vi "Main.vi"() -> ()   [LabVIEW 2022 SP3, in "Application.lvlib"]
doc: "This VI is the main application VI in the DQMH project template. This application VI is implemented as a simple state machine, which communicates with two different DQMH modules.\n_____\nBased on DQMH Project Template 7.0.1.1316."
uses:
  Application.lvlib
  Application Data--cluster.ctl
  State--enum.ctl
  <vilib>/Utility/error.llb/DialogType.ctl
  <vilib>/MakerHub/LINX/Public/Utilities/Open Local.vi
  HW-210/HW-210_dqmh.lvlib
  BME680/BME680_dqmh.lvlib
  Motor/Motor.lvlib
  <vilib>/MakerHub/LINX/LMH-LINX.lvlib
panel:
  in  "Boolean":bool
  in  "About DQMH":bool
  out "version":string
  in  "Hide BME680 Module":bool
  in  "Show BME680 Module":bool
  in  "Hide HW-210 Module":bool
  in  "Show HW-210 Module":bool
  in  "Stop HW-210 Module":bool
  in  "Stop BME680 Module":bool
  in  "Start BME680 Module":bool
  out "Active HW-210 Modules":string[](array[string])
  in  "Select HW-210 Module Instance":i32(ring)=-1 items=["All"=-1, "1"=1]
  out "BME680 Running?":bool
  out "Status":string
  # "This top-level application allows you to launch and control a singleton module, and multiple instances of a cloneable module."
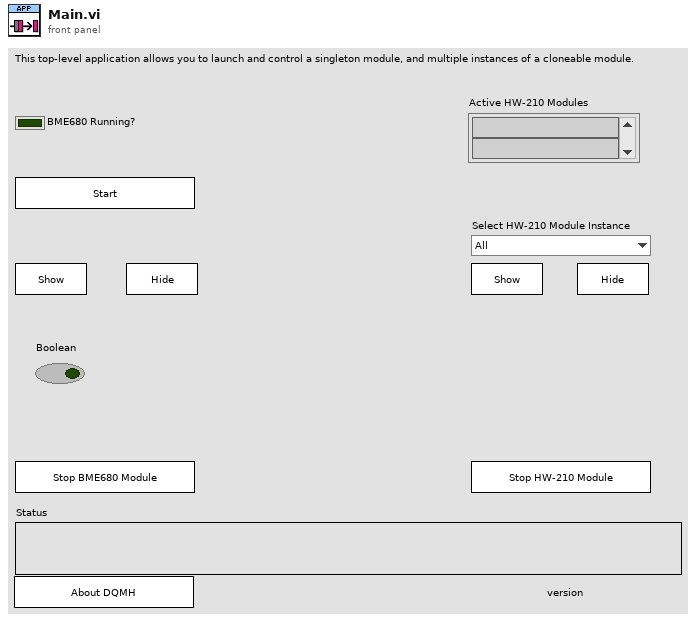
[diagram p1: front panel]
types:
  T1 = typedef "Application.lvlib/State--enum.ctl" = enum16{"Initialize", "Initialize Panel", "UI Interlocks", "Update Status", "Wait for Event", "Exit"}
  T2 = typedef "Application.lvlib/Application Data--cluster.ctl" = cluster{"Status":string, "Singleton Controls":refnum<vi>[], "Cloneable Controls":refnum<vi>[], "Module Ring Value":i32}
  T3 = typedef "Motor.lvlib/Broadcast Events--cluster.ctl" = cluster{"Module Did Init":refnum<user-event>, "Status Updated":refnum<user-event>, "Error Reported":refnum<user-event>, "Module Did Stop":refnum<user-event>, "Update Module Execution Status":refnum<user-event>, "Linx":refnum<user-event>}
  T4 = typedef "HW-210_dqmh.lvlib/Broadcast Events--cluster.ctl" = cluster{"Module Did Init":refnum<user-event>, "Status Updated":refnum<user-event>, "Error Reported":refnum<user-event>, "Module Did Stop":refnum<user-event>, "Update Module Execution Status":refnum<user-event>, "Linx":refnum<user-event>}
  T5 = typedef "BME680_dqmh.lvlib/Broadcast Events--cluster.ctl" = cluster{"Module Did Init":refnum<user-event>, "Status Updated":refnum<user-event>, "Error Reported":refnum<user-event>, "Module Did Stop":refnum<user-event>, "Update Module Execution Status":refnum<user-event>, "Linx":refnum<user-event>}
  T6 = enum8{"Enabled", "Disabled", "Disabled and Grayed Out"}
  T7 = typedef "LMH-LINX.lvlib/LINX Ref.ctl" = cluster{"IO":T8, "Interface":T9, "LINX Device Config":T10}
  T8 = typedef "LMH-LINX.lvlib/Platform.ctl" = enum16{"Remote", "Local"}
  T9 = typedef "LMH-LINX.lvlib/Interface.ctl" = enum16{"Serial", "TCP"}
  T10 = typedef "LMH-LINX.lvlib/Device.lvlib/LINX Device Config.ctl" = cluster{"Interface":T9, "COM Port":refnum<visa-resource-name>, "TCP Configuration":T11, "Device Family":u8, "Device ID":u8, "Device Name":string, "TCP Ref":refnum<k5>, "Channels":T12}
  T11 = typedef "LMH-LINX.lvlib/Device.lvlib/TCP Config.ctl" = cluster{"IP Address":string, "Port":u16}
  T12 = typedef "LMH-LINX.lvlib/Channels.ctl" = cluster{"DI":u8[], "DO":u8[], "AI":u8[], "AO":u8[], "PWM":u8[], "QE":u8[], "UART":u8[], "I2C 2":u8[], "SPI":u8[], "CAN":u8[], "Servo":u8[], "AI Ref (V)":dbl, "AI Resolution (Bits)":u8, "AO Ref (V)":dbl, "AO Resolution (Bits)":u8}
  T13 = typedef "DialogType.ctl" = u16
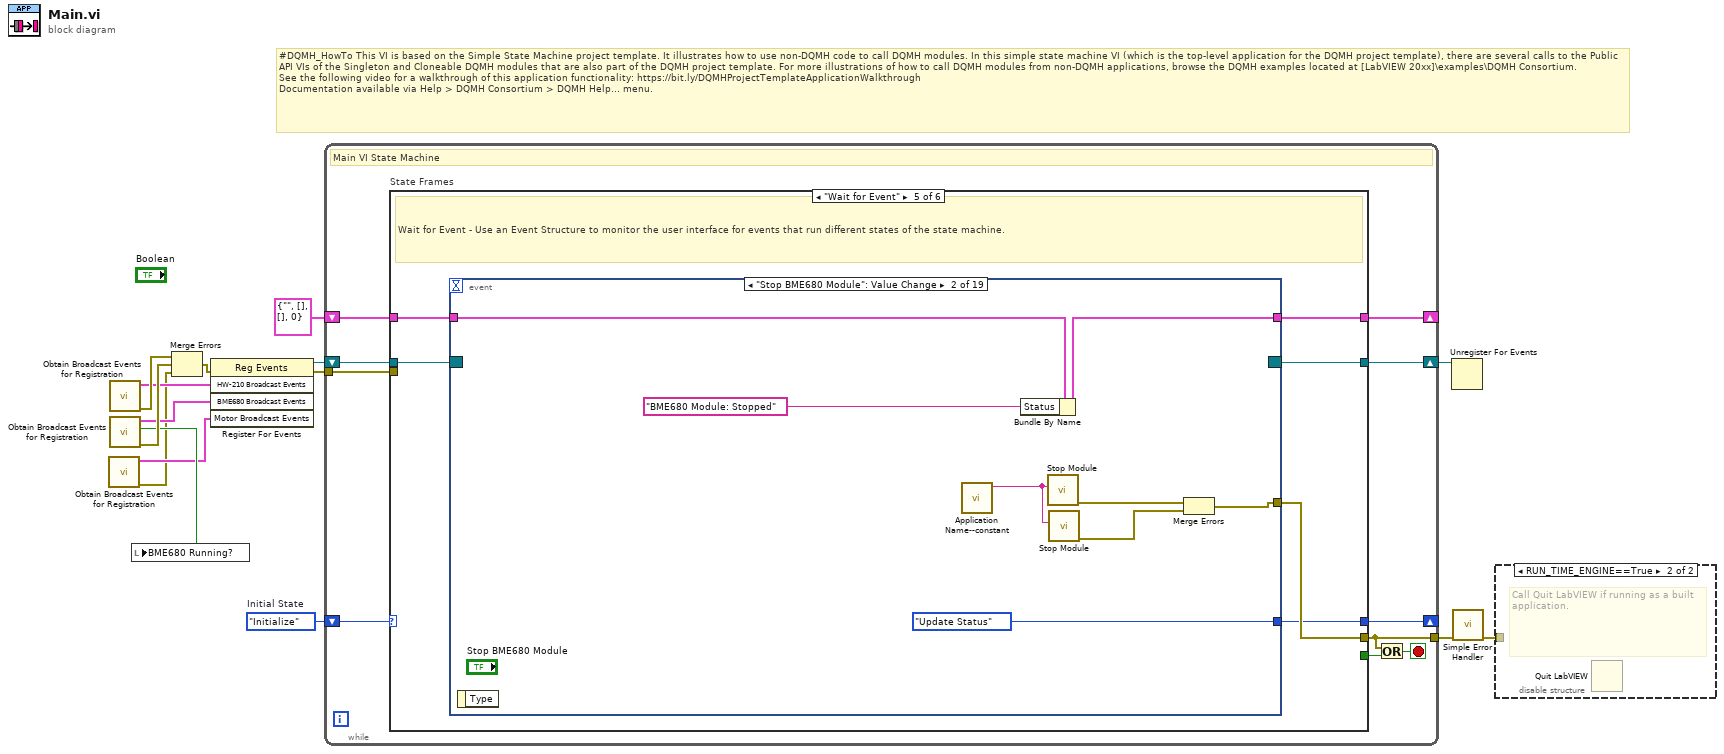
[diagram p0: block diagram]
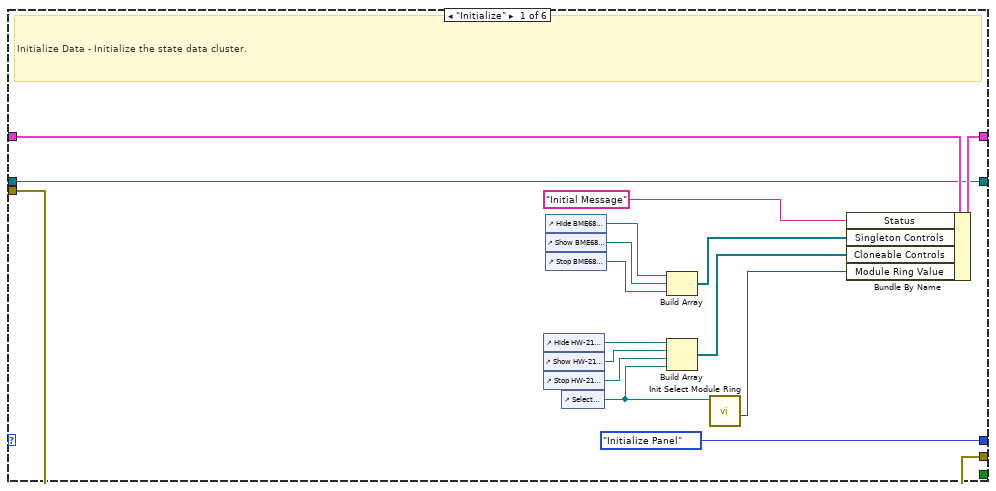
[diagram p2: hidden frame]
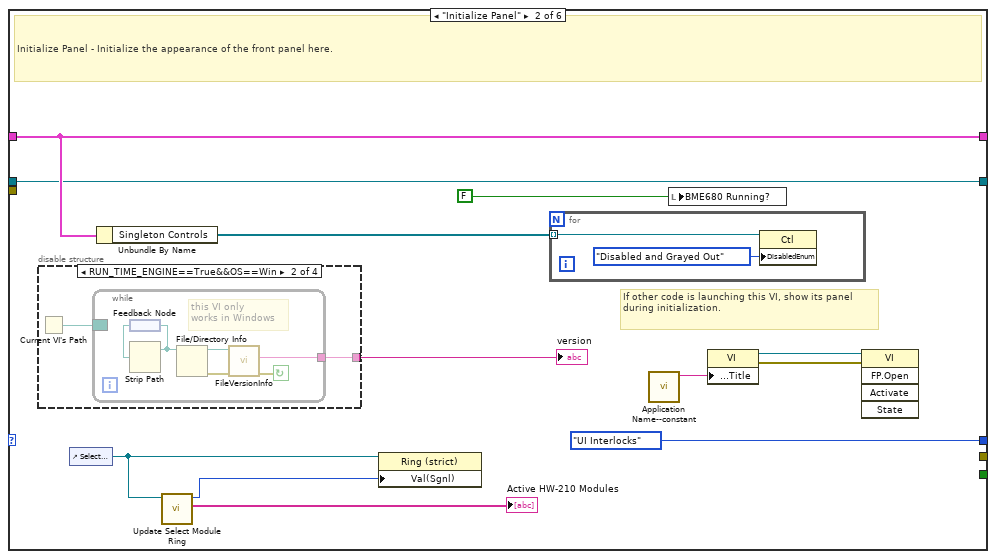
[diagram p3: hidden frame]
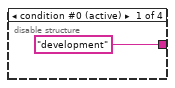
[diagram p4: hidden frame]
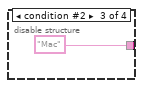
[diagram p5: hidden frame]
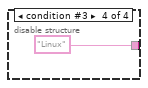
[diagram p6: hidden frame]
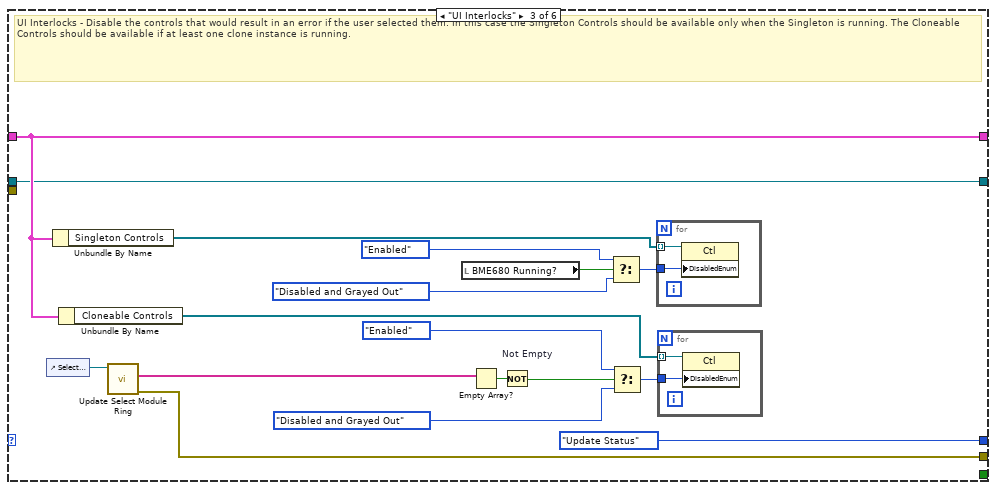
[diagram p7: hidden frame]
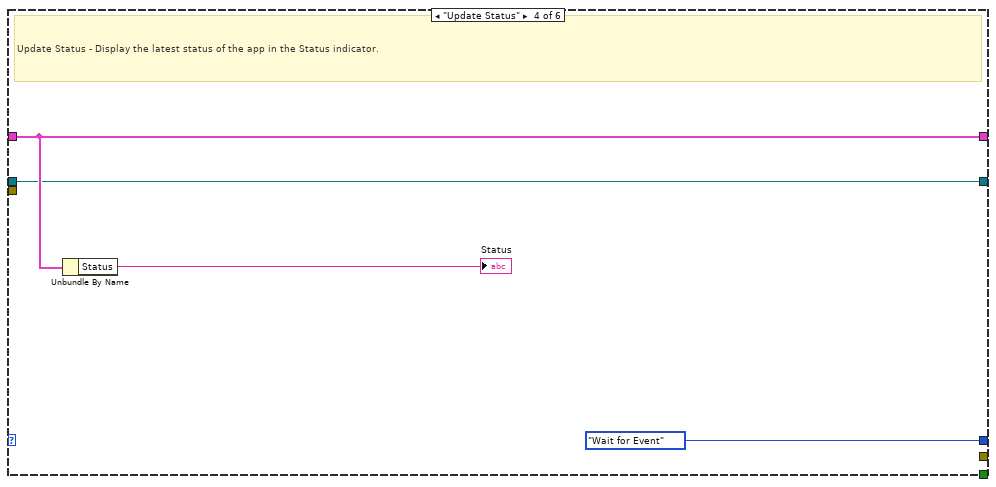
[diagram p8: hidden frame]
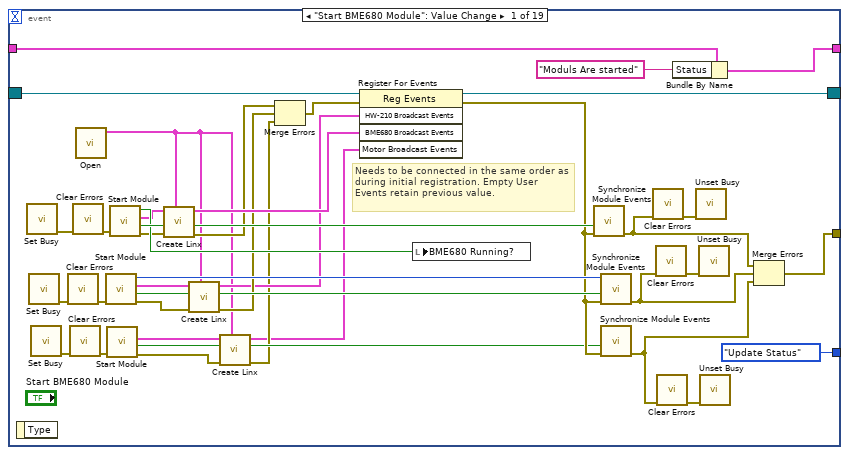
[diagram p9: hidden frame]
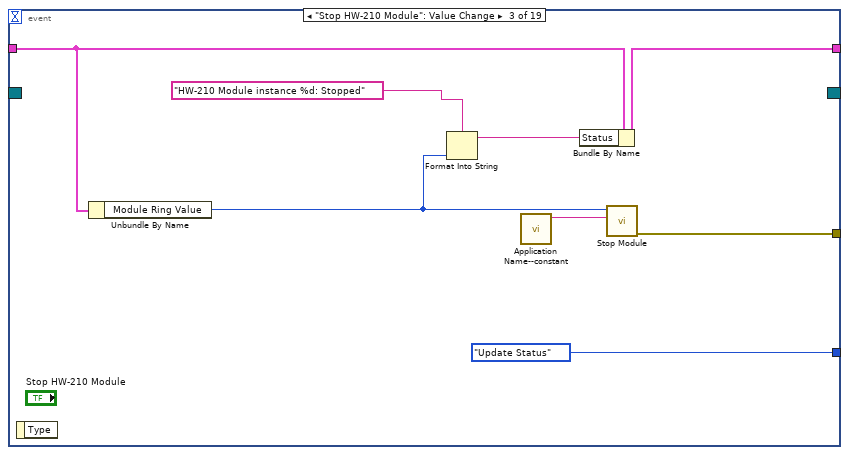
[diagram p10: hidden frame]
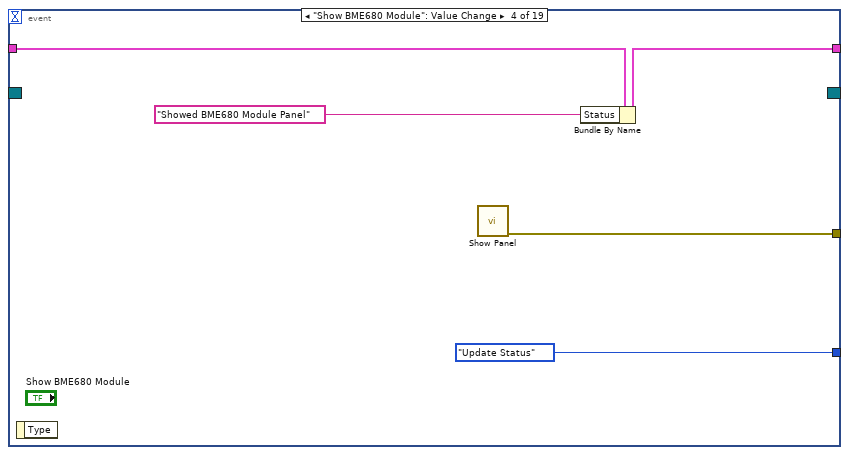
[diagram p11: hidden frame]
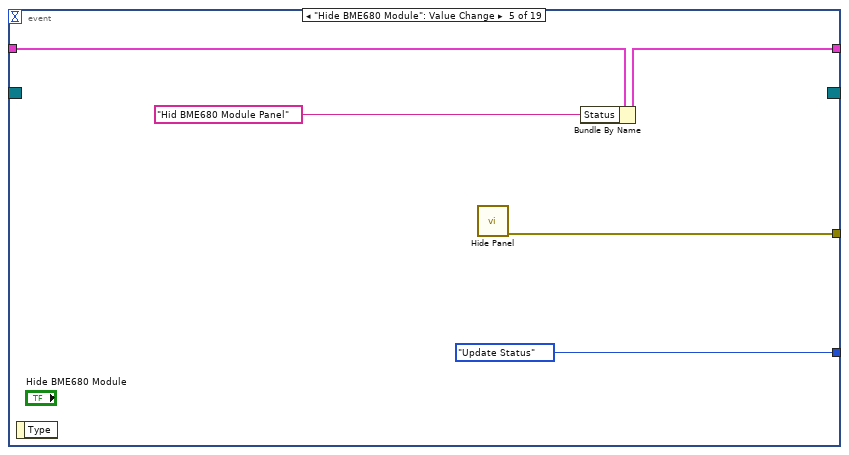
[diagram p12: hidden frame]
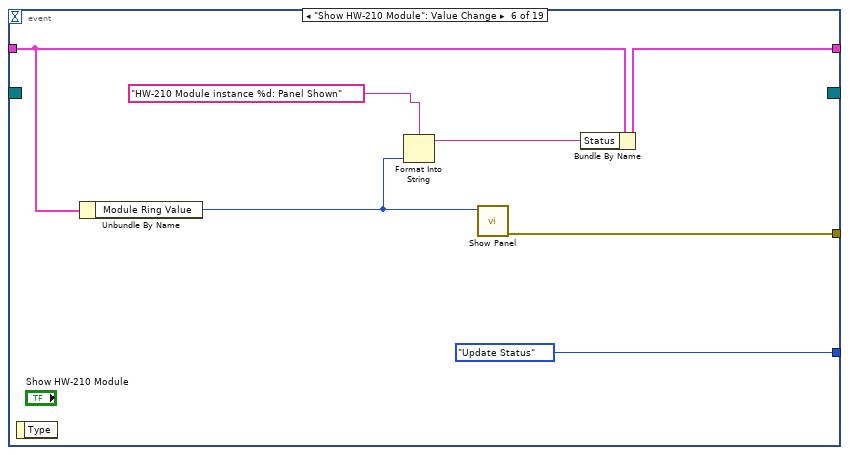
[diagram p13: hidden frame]
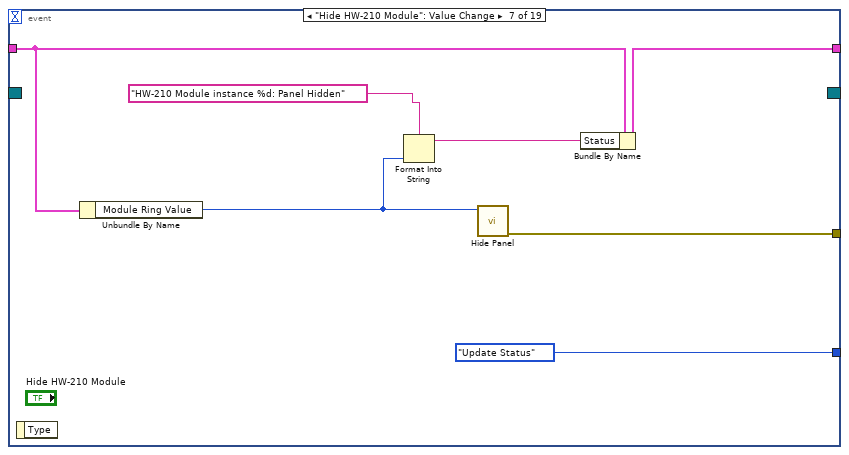
[diagram p14: hidden frame]
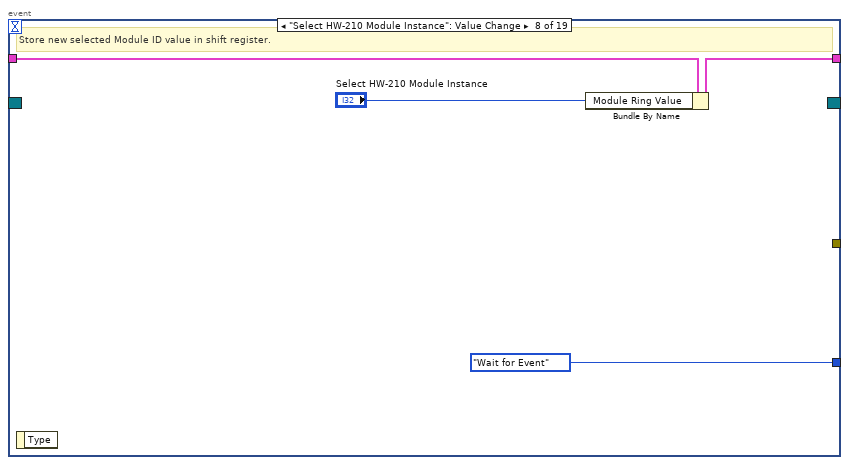
[diagram p15: hidden frame]
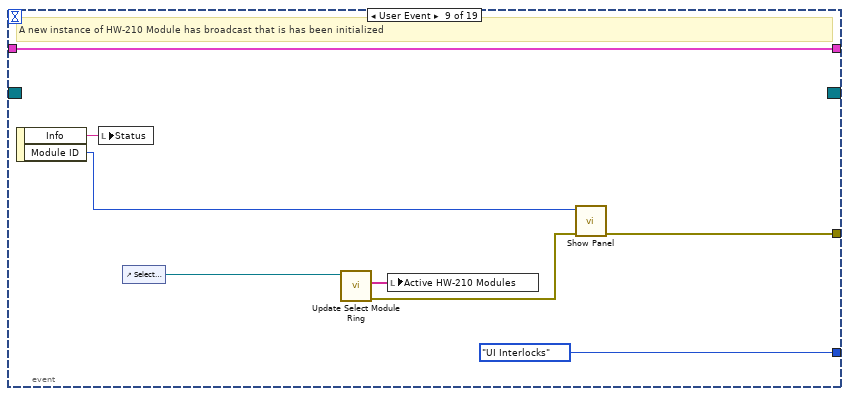
[diagram p16: hidden frame]
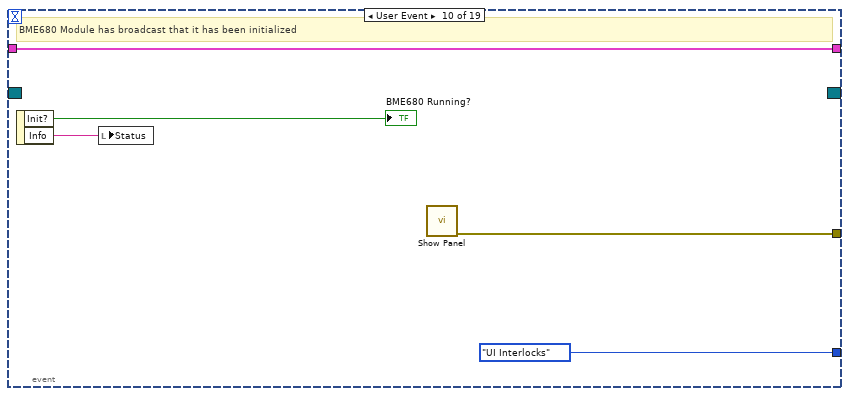
[diagram p17: hidden frame]
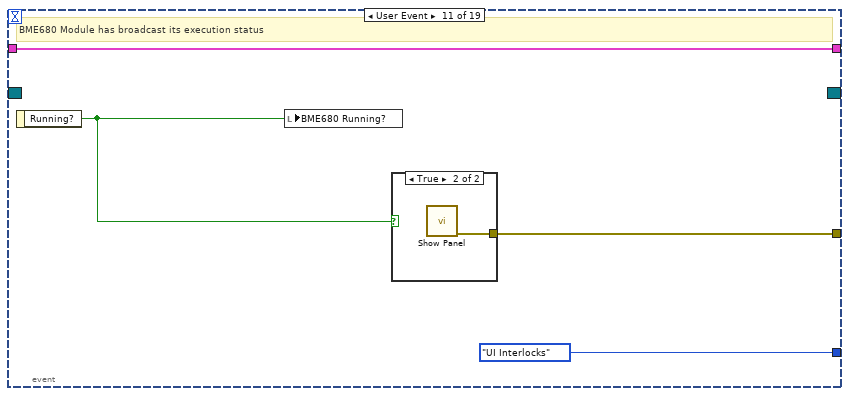
[diagram p18: hidden frame]
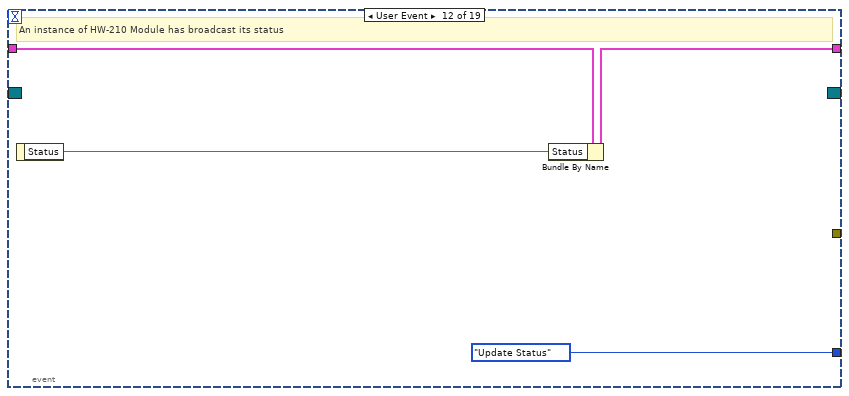
[diagram p20: hidden frame]
diagram:
  w6 = State--enum."Initialize"  # Initial State
  # "#DQMH_HowTo This VI is based on the Simple State Machine project template. It illustrates how to use non-DQMH code to call DQMH modules. In this simple state machine VI (which is the top-level application for the DQMH project template), there are several calls to the Public API VIs of the Singleton and Cloneable DQMH modules that are also part of the DQMH project template. For more illustrations of how to call DQMH modules from non-DQMH applications, browse the DQMH examples located at [LabVIEW 20xx]\\examples\\DQMH Consortium.\nSee the following video for a walkthrough of this application functionality: https://bit.ly/DQMHProjectTemplateApplicationWalkthrough\nDocumentation available via Help > DQMH Consortium > DQMH Help... menu."
  n1 = call "Obtain Broadcast Events for Registration.vi"() -> ("error out"=w1:errorcluster, "Motor Broadcast Events"=w2:T3)  [unwired: 9 in, 1 out]
  n2 = call "Obtain Broadcast Events for Registration.vi"() -> ("error out"=w11:errorcluster, "HW-210 Broadcast Events"=w8:T4)  [unwired: 9 in, 1 out]
  n3 = call "Obtain Broadcast Events for Registration.vi"() -> ("error out"=w10:errorcluster, "Already running?"=w3:bool, "BME680 Broadcast Events"=w7:T5)  [unwired: 9 in]
  n4 = local write "BME680 Running?"(w3) -> ()
  n5 = Merge Errors(w11, w10, w1) -> (w12:errorcluster)
  n6 = register-events(error in=w12, w8, w7, w2) -> (reference out=w5:refnum<event-registration>, error out=w13:errorcluster)  [unwired: 1 in]
  n7 = while {
    shift-right: [w22] -> _
    shift-left: T2 {"Status"="", "Singleton Controls"=[], "Cloneable Controls"=[], "Module Ring Value"=0} ("Data Cluster") -> [w23]
    tunnel: [w25] -> w15
    shift-right: [w18] -> _
    shift-left: w6 -> [w20]
    shift-right: [w16] -> w4
    shift-left: w5 -> [w17]
    tunnel: w13 -> [w24]
    stop <- w19 stop-if-true
    # "Main VI State Machine"
    n8 = case "State Frames" shown="\"Wait for Event\"" w20 {
      tunnel: [w41 _ w83 _ w97 w263] -> w25
      tunnel: w23 -> [w40 w50 w71 w91 w94 w260]
      tunnel: [w39 w50 w71 w91 w93 w260] -> w22
      tunnel: [_ _ _ _ _ w259] -> w21
      tunnel: [State--enum."Initialize Panel" ("State") State--enum."UI Interlocks" ("State") State--enum."Update Status" ("State") State--enum."Wait for Event" ("State") w92 State--enum."Exit" ("State")] -> w18
      tunnel: w17 -> [w26 w47 w67 w88 w96 w257]
      tunnel: [w26 w47 w67 w88 w95 w257] -> w16
      tunnel: w24 -> [w41 _ _ _ _ _]
      frame "Initialize" {
        # "Initialize Data - Initialize the state data cluster."
        n9 = control-ref of="Hide HW-210 Module"() -> (w33:refnum<vi>)
        n10 = control-ref of="Show HW-210 Module"() -> (w32:refnum<vi>)
        n11 = control-ref of="Stop HW-210 Module"() -> (w31:refnum<vi>)
        n12 = control-ref of="Hide BME680 Module"() -> (w37:refnum<vi>)
        n13 = control-ref of="Show BME680 Module"() -> (w36:refnum<vi>)
        n14 = control-ref of="Stop BME680 Module"() -> (w35:refnum<vi>)
        n15 = control-ref of="Select HW-210 Module Instance"() -> (w28:refnum<vi>)
        n16 = Build Array(w37, w36, w35) -> (w34:refnum<vi>[])
        n17 = Build Array(w33, w32, w31, w28) -> (w30:refnum<vi>[])
        n18 = call "Init Select Module Ring.vi"("Select Module Ring Ref"=w28) -> ("Module Ring Value"=w27:i32)  [unwired: 8 in, 2 out]
        n19 = Bundle By Name(cluster=w40, "Status"="Initial Message" ("Initial Message"), "Singleton Controls"=w34, "Cloneable Controls"=w30, "Module Ring Value"=w27) -> (w39:T2)
      }
      frame "Initialize Panel" {
        # "If other code is launching this VI, show its panel during initialization."
        # "Initialize Panel - Initialize the appearance of the front panel here."
        n20 = disable-structure "Conditional Disable Structure" shown="RUN_TIME_ENGINE==True&&OS==Win" {
          disable-tunnel: ["development" w55 "Mac" "Linux"] -> w44
          frame condition #0 (active) {
          }
          frame condition #1 {
            n21 = Current VI's Path() -> (path=w56:path)
            n22 = while {
              border: w56 -> [_]
              tunnel: [w57] -> w55
              stop <- w61 continue-if-true
              # "this VI only \nworks in Windows"
              n23 = feedback #1() -> (w60:path)
              n24 = Strip Path(path=w60) -> (stripped path=w59:path)  [unwired: 1 out]
              n25 = feedback-in #1(w59) -> ()
              n26 = File/Directory Info(path=w59) -> (path out=w58:path, error out=w62:errorcluster)  [unwired: 1 in, 5 out]
              n27 = call <vilib>:"FileVersionInfo.vi"("error in (no error)"=w62, "Application Path in"=w58) -> ("error out"=w61:errorcluster, "File Version Info"=w57:string)  [unwired: 6 in, 2 out]
            }
          }
          frame condition #2 {
          }
          frame condition #3 {
          }
        }
        "version" <- w44
        n28 = control-ref of="Select HW-210 Module Instance"() -> (w46:refnum<vi>)
        n29 = Unbundle By Name(w50) -> ("Singleton Controls"=w49:refnum<vi>[])
        n30 = call "Update Select Module Ring.vi"("Select Module Ring Ref"=w46) -> ("Active Modules (Array)"=→"Active HW-210 Modules":string[], "New Module Ring Value"=w45:i32)  [unwired: 8 in, 1 out]
        n31 = property on="Property Node" class="Ring (strict)"(reference=w46, "Val(Sgnl)"=w45) -> ()  [unwired: 1 in, 2 out]
        n32 = for {
          tunnel: w49 -> [w66] mode=indexing
          n33 = property on="Property Node" class="Ctl"(reference=w66, "DisabledEnum"=T6."Disabled and Grayed Out" ("Disabled")) -> ()  [unwired: 1 in, 2 out]
        }
        n34 = call "Application Name--constant.vi"() -> ("Application Name"=w43:string)  [unwired: 11 in]
        n35 = local write "BME680 Running?"(FALSE ("My Singleton Module Init?")) -> ()
        n36 = property on="Property Node" class="VI"("Front Panel.Title"=w43) -> (reference out=w42:refnum<vi>, error out=w53:errorcluster)  [unwired: 2 in]
        n37 = invoke class="VI" method="FP.Open"(reference=w42, error in=w53) -> ()  [unwired: 3 in, 5 out]
      }
      frame "UI Interlocks" {
        # "UI Interlocks - Disable the controls that would result in an error if the user selected them. In this case the Singleton Controls should be available only when the Singleton is running. The Cloneable Controls should be available if at least one clone instance is running."
        n38 = control-ref of="Select HW-210 Module Instance"() -> (w82:refnum<vi>)
        n39 = Unbundle By Name(w71) -> ("Singleton Controls"=w76:refnum<vi>[])
        n40 = Unbundle By Name(w71) -> ("Cloneable Controls"=w70:refnum<vi>[])
        n41 = call "Update Select Module Ring.vi"("Select Module Ring Ref"=w82) -> ("error out"=w83:errorcluster, "Active Modules (Array)"=w81:string[])  [unwired: 8 in, 1 out]
        n42 = local read "BME680 Running?"() -> (w75:bool)
        n43 = Empty Array?(array=w81) -> (empty?=w80:bool)
        n44 = Not "Not Empty"(x=w80) -> (.not. x?=w69:bool)
        n45 = Select(t=T6."Enabled" ("Disabled"), s=w75, f=T6."Disabled and Grayed Out" ("Disabled")) -> (s? t:f=w77:T6)
        n46 = Select(t=T6."Enabled" ("Disabled"), s=w69, f=T6."Disabled and Grayed Out" ("Disabled")) -> (s? t:f=w74:T6)
        n47 = for {
          tunnel: w76 -> [w87] mode=indexing
          tunnel: w77 -> [w86]
          n48 = property on="Property Node" class="Ctl"(reference=w87, "DisabledEnum"=w86) -> ()  [unwired: 1 in, 2 out]
        }
        n49 = for {
          tunnel: w70 -> [w85] mode=indexing
          tunnel: w74 -> [w84]
          n50 = property on="Property Node" class="Ctl"(reference=w85, "DisabledEnum"=w84) -> ()  [unwired: 1 in, 2 out]
        }
      }
      frame "Update Status" {
        # "Update Status - Display the latest status of the app in the Status indicator."
        n51 = Unbundle By Name(w91) -> ("Status"=→"Status":string)
      }
      frame "Wait for Event" {
        # "Wait for Event - Use an Event Structure to monitor the user interface for events that run different states of the state machine."
        n52 = event shown="[1] \"Stop BME680 Module\": Value Change" {
          selector: w96 -> [w132 _ _ _ _ _ _ _ _ _ _ _ _ _ _ _ _ _ _]
          dyn-events: [w131 _ _ _ _ _ _ _ _ _ _ _ _ _ _ _ _ _ _] -> w95
          timeout: _ -> [_ _ _ _ _ _ _ _ _ _ _ _ _ _ _ _ _ _ _]
          tunnel: [w118 w137 w152 w157 w162 w169 w176 _ w188 w193 w197 _ _ _ _ w239 _ _ w250] -> w97
          tunnel: [w128 w142 w149 w155 w160 w168 w175 w178 w182 w190 w196 w199 w204 w219 w228 w232 w243 w248 w252] -> w93
          tunnel: w94 -> [w129 w143 w148 w156 w161 w166 w173 w179 w182 w190 w196 w200 w205 w220 w229 w235 w244 w248 w252]
          tunnel: [State--enum."Update Status" ("State") State--enum."Update Status" ("State") State--enum."Update Status" ("State") State--enum."Update Status" ("State") State--enum."Update Status" ("State") State--enum."Update Status" ("State") State--enum."Update Status" ("State") State--enum."Wait for Event" ("State") State--enum."UI Interlocks" ("State") State--enum."UI Interlocks" ("State") State--enum."UI Interlocks" ("State") State--enum."Update Status" ("State") State--enum."Update Status" ("State") State--enum."Update Status" ("State") State--enum."Update Status" ("State") State--enum."UI Interlocks" ("State") State--enum."UI Interlocks" ("State") State--enum."Exit" ("State") State--enum."Wait for Event" ("State")] -> w92
          event "Start BME680 Module": Value Change {
            # "Needs to be connected in the same order as during initial registration. Empty User Events retain previous value."
            n53 = event-data() -> ()  [unwired: 1 in, 1 out]
            n54 = call <vilib>:"Set Busy.vi"() -> ("error out"=w135:errorcluster)  [unwired: 10 in, 1 out]
            n55 = call <vilib>:"Set Busy.vi"() -> ("error out"=w124:errorcluster)  [unwired: 10 in, 1 out]
            n56 = call <vilib>:"Set Busy.vi"() -> ("error out"=w117:errorcluster)  [unwired: 10 in, 1 out]
            n57 = call <vilib>:"Clear Errors.vi"("error in (no error)"=w124) -> ("error out"=w125:errorcluster)  [unwired: 5 in, 1 out]
            n58 = call <vilib>:"Clear Errors.vi"("error in (no error)"=w117) -> ("error out"=w116:errorcluster)  [unwired: 5 in, 1 out]
            n59 = call <vilib>:"Clear Errors.vi"("error in (no error)"=w135) -> ("error out"=w136:errorcluster)  [unwired: 5 in, 1 out]
            n60 = call-poly <vilib>:"Open.vi"() -> ("LINX Resource"=w98:T7)  [unwired: 9 in, 2 out]
            n61 = call "Start Module.vi"("error in"=w125) -> ("error out"=w105:errorcluster, "Wait for Event Sync?"=w122:bool, "HW-210 Broadcast Events"=w106:T4, "Module ID"=w121:i32)  [unwired: 7 in]
            n62 = call "Start Module.vi"("error in"=w116) -> ("error out"=w102:errorcluster, "Wait for Event Sync?"=w114:bool, "Motor Broadcast Events"=w101:T3)  [unwired: 7 in, 1 out]
            n63 = call "Start Module.vi"("error in"=w136) -> ("error out"=w110:errorcluster, "Wait for Event Sync?"=w133:bool, "BME680 Broadcast Events"=w109:T5, "Module Was Already Running?"=w126:bool)  [unwired: 7 in]
            n64 = call "Create Linx.vi"("LINX Resource"=w98, "error in (no error)"=w110, "Broadcast Events In"=w109) -> ("error out"=w107:errorcluster, "Broadcast Events Out"=w108:T5)  [unwired: 7 in]
            n65 = call "Create Linx.vi"("LINX Resource"=w98, "error in (no error)"=w105, "Broadcast Events In"=w106) -> ("error out"=w104:errorcluster, "Broadcast Events Out"=w103:T4)  [unwired: 7 in]
            n66 = call "Create Linx.vi"("LINX Resource"=w98, "error in (no error)"=w102, "Broadcast Events In"=w101) -> ("error out"=w100:errorcluster, "Broadcast Events Out"=w99:T3)  [unwired: 7 in]
            n67 = Merge Errors(w107, w104, w100) -> (w120:errorcluster)
            n68 = register-events(reference=w132, error in=w120, w103, w108, w99) -> (reference out=w131:refnum<event-registration>, error out=w115:errorcluster)
            n69 = local write "BME680 Running?"(w126) -> ()
            n70 = call "Synchronize Module Events.vi"("error in"=w115, "Wait for Event Sync?"=w133) -> ("error out"=w119:errorcluster)  [unwired: 9 in]
            n71 = call "Synchronize Module Events.vi"("error in"=w115, "Wait for Event Sync?"=w122, "Module ID in"=w121) -> ("error out"=w113:errorcluster)  [unwired: 7 in, 1 out]
            n72 = call "Synchronize Module Events.vi"("error in"=w115, "Wait for Event Sync?"=w114) -> ("error out"=w111:errorcluster)  [unwired: 9 in]
            n73 = call <vilib>:"Clear Errors.vi"("error in (no error)"=w119) -> ("error out"=w134:errorcluster)  [unwired: 5 in, 1 out]
            n74 = call <vilib>:"Clear Errors.vi"("error in (no error)"=w113) -> ("error out"=w123:errorcluster)  [unwired: 5 in, 1 out]
            n75 = call <vilib>:"Clear Errors.vi"("error in (no error)"=w111) -> ("error out"=w112:errorcluster)  [unwired: 5 in, 1 out]
            n76 = Bundle By Name(cluster=w129, "Status"="Moduls Are started") -> (w128:T2)
            n77 = call <vilib>:"Unset Busy.vi"("error in (no error)"=w134) -> ()  [unwired: 10 in, 1 out]
            n78 = call <vilib>:"Unset Busy.vi"("error in (no error)"=w123) -> ()  [unwired: 10 in, 1 out]
            n79 = call <vilib>:"Unset Busy.vi"("error in (no error)"=w112) -> ()  [unwired: 10 in, 1 out]
            n80 = Merge Errors(w119, w113, w111) -> (w118:errorcluster)
          }
          event "Stop BME680 Module": Value Change {
            n81 = event-data() -> ()  [unwired: 1 in, 1 out]
            n82 = call "Application Name--constant.vi"() -> ("Application Name"=w140:string)  [unwired: 11 in]
            n83 = Bundle By Name(cluster=w143, "Status"="BME680 Module: Stopped" ("Message")) -> (w142:T2)
            n84 = call "Stop Module.vi"("Origin"=w140) -> ("error out"=w139:errorcluster)  [unwired: 10 in]
            n85 = call "Stop Module.vi"("Origin"=w140) -> ("error out"=w138:errorcluster)  [unwired: 10 in]
            n86 = Merge Errors(w139, w138) -> (w137:errorcluster)
          }
          event "Stop HW-210 Module": Value Change {
            n87 = event-data() -> ()  [unwired: 1 in, 1 out]
            n88 = Unbundle By Name(w148) -> ("Module Ring Value"=w145:i32)
            n89 = Format Into String(format string="HW-210 Module instance %d: Stopped" ("Message"), w145) -> (resulting string=w146:string)  [unwired: 2 in, 1 out]
            n90 = call "Application Name--constant.vi"() -> ("Application Name"=w150:string)  [unwired: 11 in]
            n91 = Bundle By Name(cluster=w148, "Status"=w146) -> (w149:T2)
            n92 = call "Stop Module.vi"("Origin"=w150, "Module ID"=w145) -> ("error out"=w152:errorcluster)  [unwired: 9 in]
          }
          event "Show BME680 Module": Value Change {
            n93 = event-data() -> ()  [unwired: 1 in, 1 out]
            n94 = call "Show Panel.vi"() -> ("error out"=w157:errorcluster)  [unwired: 11 in]
            n95 = Bundle By Name(cluster=w156, "Status"="Showed BME680 Module Panel" ("Message")) -> (w155:T2)
          }
          event "Hide BME680 Module": Value Change {
            n96 = event-data() -> ()  [unwired: 1 in, 1 out]
            n97 = call "Hide Panel.vi"() -> ("error out"=w162:errorcluster)  [unwired: 11 in]
            n98 = Bundle By Name(cluster=w161, "Status"="Hid BME680 Module Panel" ("Message")) -> (w160:T2)
          }
          event "Show HW-210 Module": Value Change {
            n99 = event-data() -> ()  [unwired: 1 in, 1 out]
            n100 = Unbundle By Name(w166) -> ("Module Ring Value"=w164:i32)
            n101 = Format Into String(format string="HW-210 Module instance %d: Panel Shown" ("Message"), w164) -> (resulting string=w163:string)  [unwired: 2 in, 1 out]
            n102 = call "Show Panel.vi"("Module ID"=w164) -> ("error out"=w169:errorcluster)  [unwired: 10 in]
            n103 = Bundle By Name(cluster=w166, "Status"=w163) -> (w168:T2)
          }
          event "Hide HW-210 Module": Value Change {
            n104 = event-data() -> ()  [unwired: 1 in, 1 out]
            n105 = Unbundle By Name(w173) -> ("Module Ring Value"=w171:i32)
            n106 = Format Into String(format string="HW-210 Module instance %d: Panel Hidden" ("Message"), w171) -> (resulting string=w170:string)  [unwired: 2 in, 1 out]
            n107 = call "Hide Panel.vi"("Module ID"=w171) -> ("error out"=w176:errorcluster)  [unwired: 10 in]
            n108 = Bundle By Name(cluster=w173, "Status"=w170) -> (w175:T2)
          }
          event "Select HW-210 Module Instance": Value Change {
            # "Store new selected Module ID value in shift register."
            n109 = event-data() -> ()  [unwired: 1 in, 1 out]
            n110 = Bundle By Name(cluster=w179, "Module Ring Value"="Select HW-210 Module Instance") -> (w178:T2)
          }
          event User Event {
            # "A new instance of HW-210 Module has broadcast that is has been initialized"
            n111 = event-data() -> ("Info"=w186:string, "Module ID"=w181:i32)  [unwired: 1 in]
            n112 = local write "Status"(w186) -> ()
            n113 = control-ref of="Select HW-210 Module Instance"() -> (w185:refnum<vi>)
            n114 = call "Update Select Module Ring.vi"("Select Module Ring Ref"=w185) -> ("error out"=w187:errorcluster, "Active Modules (Array)"=w184:string[])  [unwired: 8 in, 1 out]
            n115 = local write "Active HW-210 Modules"(w184) -> ()
            n116 = call "Show Panel.vi"("error in"=w187, "Module ID"=w181) -> ("error out"=w188:errorcluster)  [unwired: 9 in]
          }
          event User Event {
            # "BME680 Module has broadcast that it has been initialized"
            n117 = event-data() -> ("Init?"=→"BME680 Running?":bool, "Info"=w192:string)  [unwired: 1 in]
            n118 = local write "Status"(w192) -> ()
            n119 = call "Show Panel.vi"() -> ("error out"=w193:errorcluster)  [unwired: 11 in]
          }
          event User Event {
            # "BME680 Module has broadcast its execution status"
            n120 = event-data() -> ("Running?"=w194:bool)  [unwired: 1 in]
            n121 = local write "BME680 Running?"(w194) -> ()
            n122 = case shown="True" w194 {
              tunnel: [_ w198] -> w197
              frame False {
              }
              frame True {
                n123 = call "Show Panel.vi"() -> ("error out"=w198:errorcluster)  [unwired: 11 in]
              }
            }
          }
          event User Event {
            # "An instance of HW-210 Module has broadcast its status"
            n124 = event-data() -> ("Status"=w202:string)  [unwired: 1 in]
            n125 = Bundle By Name(cluster=w200, "Status"=w202) -> (w199:T2)
          }
          event User Event {
            # "BME680 Module has broadcast its status"
            n126 = event-data() -> ("Status"=w206:string)  [unwired: 1 in]
            n127 = Bundle By Name(cluster=w205, "Status"=w206) -> (w204:T2)
          }
          event User Event {
            w211 = T13 0 items=["no dialog", "OK message", "continue or stop message", "OK message + warnings", "continue/stop + warnings"] ("type of dialog (OK msg:1)")
            # "HW-210 Module had an error"
            n128 = event-data() -> ("Module Name"=w208:string, "Additional Information"=w209:string, "Error"=w210:errorcluster)  [unwired: 1 in]
            n129 = call <vilib>:"Space Constant.vi"() -> ("String"=w215:string)
            n130 = call <vilib>:"Simple Error Handler.vi"("type of dialog (OK msg:1)"=w211, "error in (no error)"=w210) -> ("message"=w212:string)  [unwired: 3 in, 4 out]
            n131 = call <vilib>:"Search and Replace Pattern.vi"("string"=w212, "regular expression (\"\")"="[\\r\\n]" ("regular expression (\"\")"), "replace string (\"\")"=w215, "replace all? (F)"=TRUE ("replace all CR/LF with spaces")) -> ("result string"=w213:string)  [unwired: 1 in, 1 out]
            n132 = Format Into String(format string="%s: %s Additional Information: %s", w208, w213, w209) -> (resulting string=w207:string)  [unwired: 2 in, 1 out]
            n133 = Bundle By Name(cluster=w220, "Status"=w207) -> (w219:T2)
          }
          event User Event {
            # "BME680 Module had an error"
            n134 = event-data() -> ("Module Name"=w222:string, "Additional Information"=w226:string, "Error"=w230:errorcluster)  [unwired: 1 in]
            n135 = Unbundle By Name(w230) -> ("code"=w221:i32, "source"=w225:string)
            n136 = Format Into String(format string="Error code %d Module: %s  Additional Information: %s\nSource: %s", w221, w222, w226, w225) -> (resulting string=w223:string)  [unwired: 2 in, 1 out]
            n137 = Bundle By Name(cluster=w229, "Status"=w223) -> (w228:T2)
          }
          event User Event {
            n138 = event-data() -> ("Origin"=w234:string)  [unwired: 1 in]
            n139 = Bundle By Name(cluster=w235, "Status"=w234) -> (w233:T2)
            n140 = control-ref of="Select HW-210 Module Instance"() -> (w238:refnum<vi>)
            n141 = call "Update Select Module Ring.vi"("Select Module Ring Ref"=w238) -> ("error out"=w239:errorcluster, "Active Modules (Array)"=w237:string[], "New Module Ring Value"=w231:i32)  [unwired: 8 in]
            n142 = Bundle By Name(cluster=w233, "Module Ring Value"=w231) -> (w232:T2)
            n143 = local write "Active HW-210 Modules"(w237) -> ()
          }
          event User Event {
            n144 = event-data() -> ("Origin"=w241:string)  [unwired: 1 in]
            n145 = local write "BME680 Running?"(FALSE ("My Singleton Module Init?")) -> ()
            n146 = Concatenate Strings(w241, " Did Stop.") -> (w240:string)
            n147 = Bundle By Name(cluster=w244, "Status"=w240) -> (w243:T2)
          }
          event Panel Close? {
            # "Go to the 'Exit' state if the user tries to close the panel."
            n148 = event-data() -> ()  [unwired: 1 in, 1 out]
            n149 = event-data ("Event Filter Node")("Discard?"=TRUE) -> ()  [unwired: 1 in, 1 out]
          }
          event "About DQMH": Value Change {
            # "Display DQMH About Box"
            n150 = event-data() -> ()  [unwired: 1 in, 1 out]
            n151 = call <vilib>:"DQMH_About Box.vi"() -> ("error out"=w250:errorcluster)  [unwired: 11 in]
          }
        }
      }
      frame "Exit" {
        w255 = TRUE  # Wait for Module to stop?
        w259 = TRUE  # Stop the VI
        # "Stop all modules launched"
        # "Exit - Exit the application."
        n152 = call "Application Name--constant.vi"() -> ("Application Name"=w254:string)  [unwired: 11 in]
        n153 = call "Stop Module.vi"("Wait for Module to stop? (F)"=w255, "Origin"=w254, "Module ID"=-1) -> ("error out"=w261:errorcluster)  [unwired: 8 in]
        n154 = call "Stop Module.vi"("Wait for Module to Stop? (F)"=w255, "Origin"=w254) -> ("error out"=w262:errorcluster)  [unwired: 9 in]
        n155 = call "Stop Module.vi"("Origin"=w254) -> ("error out"=w253:errorcluster)  [unwired: 10 in]
        n156 = Merge Errors(w261, w262, w253) -> (w263:errorcluster)
      }
    }
    n157 = Or(x=w25, y=w21) -> (x .or. y?=w19:bool)
  }
  n158 = Unregister For Events(event registration refnum=w4) -> ()  [unwired: 1 in, 1 out]
  n159 = call <vilib>:"Simple Error Handler.vi"("error in (no error)"=w15) -> ("error out"=w14:errorcluster)  [unwired: 4 in, 4 out]
  n160 = disable-structure "Conditional Disable Structure" shown="RUN_TIME_ENGINE==True" {
    disable-tunnel: w14 -> [_ _]
    frame condition #0 (active) {
    }
    frame condition #1 {
      # "Call Quit LabVIEW if running as a built application."
      n161 = Quit LabVIEW() -> ()  [unwired: 1 in]
    }
  }
